vi "CommunicationFormat_GetHeaderLength.vi"(8 "error in (no error)":errorcluster, 11 "OXYGEN Ref In":refnum<visa-resource-name>) -> (0 "error out":errorcluster, 1 "communication_data":T1, 2 "Long Communication Header?":bool, 3 "OXYGEN Ref Out":refnum<visa-resource-name>)   [LabVIEW 2020, in "OXYGEN_Datastream.lvlib"]
doc: "Queries the setting, whether the response header is short- or long form."
uses:
  OXYGEN_Datastream.lvlib
  TypeDefs/Cluster_RawCommData.ctl
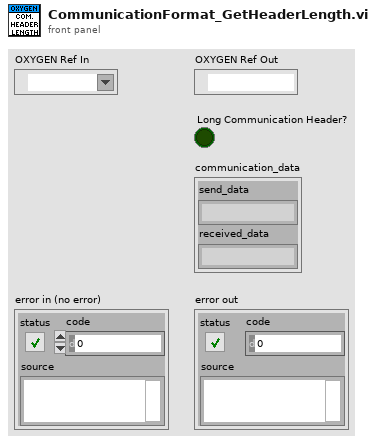
[diagram p1: front panel]
types:
  T1 = typedef "OXYGEN_Datastream.lvlib/Cluster_RawCommData.ctl" = cluster{"send_data":string, "received_data":string}
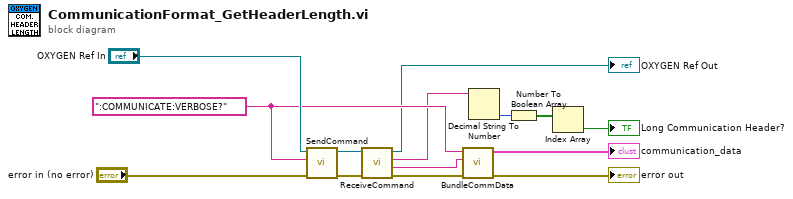
[diagram p0: block diagram]
diagram:
  w10 = ":COMMUNICATE:VERBOSE?"
  n1 = call "SendCommand.vi"("error in (no error)"="error in (no error)", "String to Send"=w10, "OXY_SCPI Reseource In"="OXYGEN Ref In") -> ("error out"=w9:errorcluster, "OXY_SCPI Reseource Out"=w7:refnum<visa-resource-name>)  [unwired: 7 in]
  n2 = call "ReceiveCommand.vi"("error in (no error)"=w9, "OXY_SCPI Reseource In"=w7) -> ("error out"=w8:errorcluster, "received Data with Header"=w1:string, "received Data"=w3:string, "OXY_SCPI Reseource Out"=→"OXYGEN Ref Out":refnum<visa-resource-name>)  [unwired: 6 in]
  n3 = call "BundleCommData.vi"("error in (no error)"=w8, "received_data"=w1, "send_data"=w10) -> ("error out"=→"error out":errorcluster, "communication_data"=→"communication_data":T1)  [unwired: 7 in]
  n4 = Decimal String To Number(string=w3) -> (number=w5:i32)  [unwired: 2 in, 1 out]
  n5 = Number To Boolean Array(number=w5) -> (Boolean array=w4:bool[])
  n6 = Index Array(array=w4) -> (element=→"Long Communication Header?":bool)  [unwired: 1 in]
